vi "QueueRepo.vi"(7 "Action":T1, 8 "error in (no error)":errorcluster, 9 "Event?":bool, 11 "Name":string) -> (0 "error out":errorcluster, 1 "Event?":bool, 2 "queue out":refnum<queue>, 3 "Names":string[](array[string]))   [LabVIEW 2017, in "Communication.lvlib"]
uses:
  Communication.lvlib
  SubVIs/QueueRepo.Action.ctl
  SubVIs/MsgData.ctl
  SubVIs/MsgAck.ctl
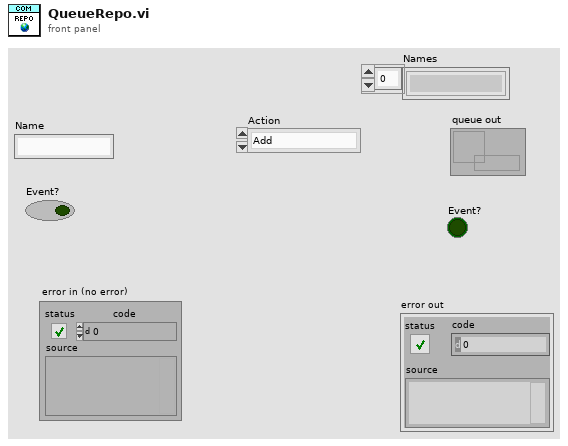
[diagram p1: front panel]
types:
  T1 = typedef "Communication.lvlib/QueueRepo.Action.ctl" = enum16{"Add", "Get", "Destroy", "Get All", "Clear"}
  T2 = typedef "Communication.lvlib/MsgData.ctl" = cluster{"Msg":string, "Data":variant, "Ack":refnum<notifier>}
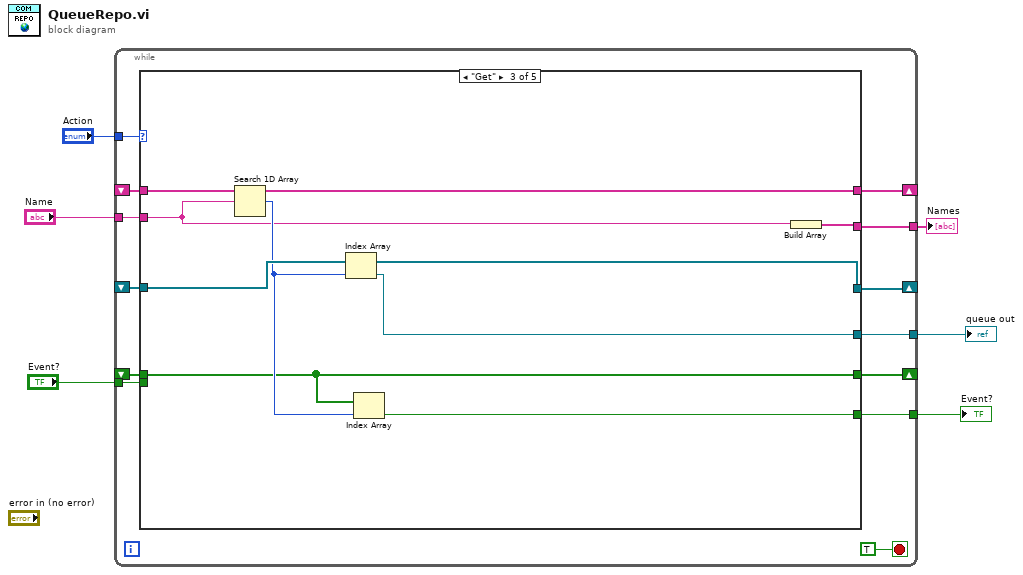
[diagram p0: block diagram]
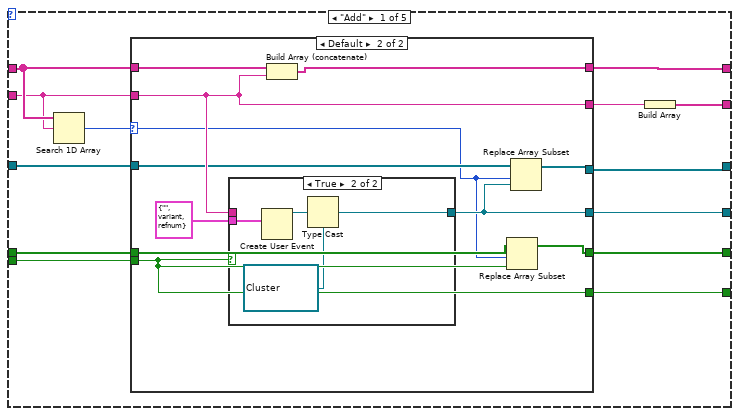
[diagram p2: hidden frame]
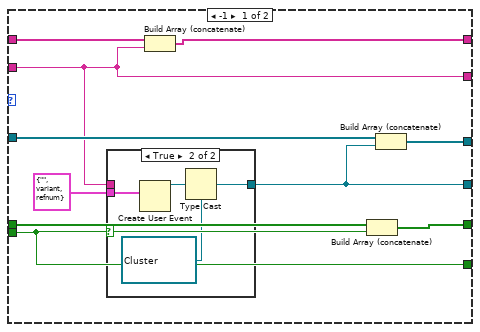
[diagram p3: hidden frame]
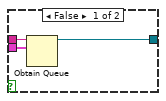
[diagram p4: hidden frame]
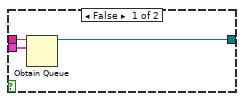
[diagram p5: hidden frame]
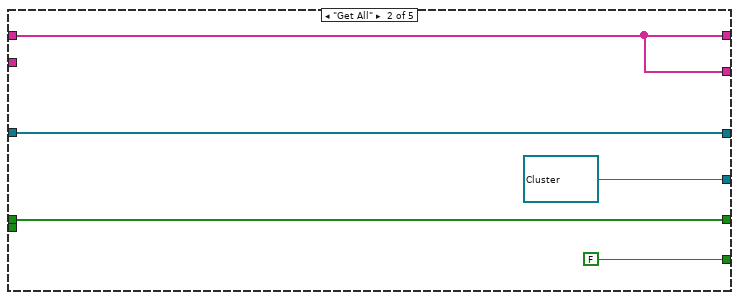
[diagram p6: hidden frame]
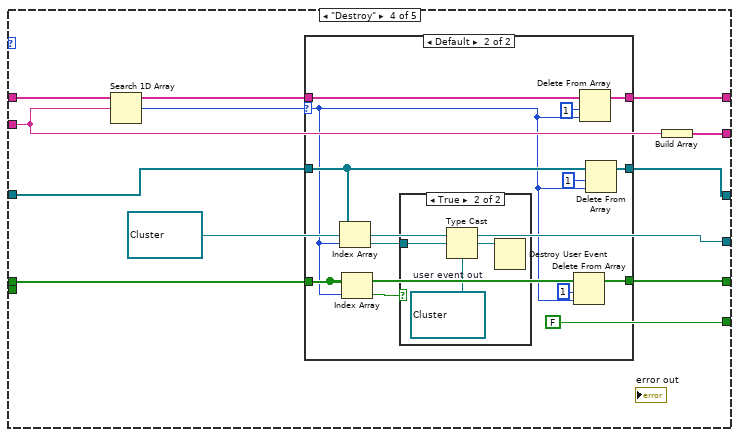
[diagram p7: hidden frame]
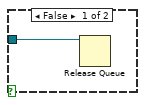
[diagram p9: hidden frame]
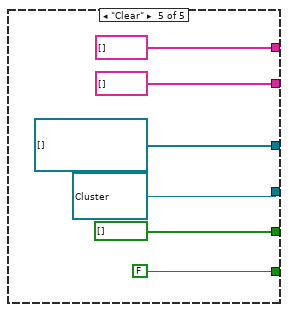
[diagram p10: hidden frame]
diagram:
  n1 = while {
    tunnel: "Action" -> [w19]
    tunnel: "Name" -> [w18]
    shift-right: [w16] -> _
    shift-left: _ -> [w15]
    shift-right: [w14] -> _
    shift-left: _ -> [w13]
    tunnel: [w12] -> w4
    tunnel: "Event?" -> [w11]
    shift-right: [w10] -> _
    shift-left: _ -> [w9]
    tunnel: [w8] -> w2
    tunnel: [w7] -> w1
    stop <- TRUE stop-if-true
    n2 = case shown="\"Get\"" w19 {
      tunnel: w18 -> [w30 _ w73 w84 _]
      tunnel: [w32 w71 w78 w81 string[] []] -> w16
      tunnel: w15 -> [w31 w71 w78 w82 _]
      tunnel: [w29 w72 w79 w90 refnum<queue>[] []] -> w14
      tunnel: w13 -> [w28 w72 w79 w91 _]
      tunnel: [w27 refnum<queue> refnum ("queue out") w80 refnum<queue> refnum ("queue out") refnum<queue> refnum ("queue out")] -> w12
      tunnel: w11 -> [w26 _ _ _ _]
      tunnel: [w25 w69 w76 w86 bool[] []] -> w10
      tunnel: w9 -> [w24 w69 w76 w87 _]
      tunnel: [w23 FALSE ("Event?") w75 FALSE FALSE ("Event?")] -> w8
      tunnel: [w21 w71 w74 w83 string[] []] -> w7
      frame "Add" {
        n3 = Search 1D Array(1D array=w31, element=w30) -> (index of element=w20:i32)  [unwired: 1 in]
        n4 = case shown="Default" w20 {
          selector: w20 -> [_ w51]
          tunnel: [w33 w57] -> w32
          tunnel: w31 -> [w42 w60]
          tunnel: w30 -> [w34 w58]
          tunnel: [w40 w54] -> w29
          tunnel: w28 -> [w39 w56]
          tunnel: [w38 w55] -> w27
          tunnel: w26 -> [w35 w52]
          tunnel: [w37 w50] -> w25
          tunnel: w24 -> [w36 w53]
          tunnel: [w35 w52] -> w23
          tunnel: [w34 w58] -> w22
          frame -1 {
            n5 = case shown="True" w35 {
              tunnel: w34 -> [w45 _]
              tunnel: T2 {"Msg"="", "Data"=variant, "Ack"=refnum} ("Cluster") -> [w44 w49]
              tunnel: [w43 w46] -> w38
              frame False {
                n6 = Obtain Queue(name (unnamed)=w45, element data type=w44) -> (queue out=w43:refnum<queue>)  [unwired: 3 in, 2 out]
              }
              frame True {
                n7 = Create User Event(user event datatype=w49) -> (user event=w48:refnum<user-event>)  [unwired: 1 in, 1 out]
                n8 = Type Cast(type=refnum<queue> refnum ("queue out"), x=w48) -> (*(type *) &x=w46:refnum<queue>)
              }
            }
            n9 = Build Array (concatenate)(w42, w34) -> (w33:string[])
            n10 = Build Array (concatenate)(w36, w35) -> (w37:bool[])
            n11 = Build Array (concatenate)(w39, w38) -> (w40:refnum<queue>[])
          }
          frame Default {
            n12 = case shown="True" w52 {
              tunnel: w58 -> [w63 _]
              tunnel: T2 {"Msg"="", "Data"=variant, "Ack"=refnum} ("Cluster") -> [w62 w67]
              tunnel: [w61 w64] -> w55
              frame False {
                n13 = Obtain Queue(name (unnamed)=w63, element data type=w62) -> (queue out=w61:refnum<queue>)  [unwired: 3 in, 2 out]
              }
              frame True {
                n14 = Create User Event(user event datatype=w67) -> (user event=w66:refnum<user-event>)  [unwired: 1 in, 1 out]
                n15 = Type Cast(type=refnum<queue> refnum ("queue out"), x=w66) -> (*(type *) &x=w64:refnum<queue>)
              }
            }
            n16 = Build Array (concatenate)(w60, w58) -> (w57:string[])
            n17 = Replace Array Subset(array=w53, new element=w52, index=w51) -> (w50:bool[])
            n18 = Replace Array Subset(array=w56, new element=w55, index=w51) -> (w54:refnum<queue>[])
          }
        }
        n19 = Build Array(w22) -> (w21:string[])
      }
      frame "Get All" {
      }
      frame "Get" {
        n20 = Search 1D Array(1D array=w78, element=w73) -> (index of element=w77:i32)  [unwired: 1 in]
        n21 = Index Array(array=w79, index=w77) -> (element=w80:refnum<queue>)
        n22 = Index Array(array=w76, index=w77) -> (element=w75:bool)
        n23 = Build Array(w73) -> (w74:string[])
      }
      frame "Destroy" {
        n24 = Search 1D Array(1D array=w82, element=w84) -> (index of element=w88:i32)  [unwired: 1 in]
        n25 = case shown="Default" w88 {
          selector: w88 -> [_ w95]
          tunnel: w91 -> [w94 w105]
          tunnel: [w94 w104] -> w90
          tunnel: w87 -> [w93 w101]
          tunnel: [w93 w100] -> w86
          tunnel: w82 -> [w92 w98]
          tunnel: [w92 w97] -> w81
          frame -1 {
          }
          frame Default {
            n26 = Index Array(array=w105, index=w95) -> (element=w106:refnum<queue>)
            n27 = Index Array(array=w101, index=w95) -> (element=w102:bool)
            n28 = case shown="True" w102 {
              tunnel: w106 -> [w107 w110]
              frame False {
                n29 = Release Queue(queue=w107) -> ()  [unwired: 2 in, 3 out]
              }
              frame True {
                w109 = refnum<user-event> refnum  # user event out
                n30 = Type Cast(type=w109, x=w110) -> (*(type *) &x=w108:refnum<user-event>)
                n31 = Destroy User Event(user event=w108) -> ()  [unwired: 1 in, 1 out]
              }
            }
            n32 = Delete From Array(array=w101, length=1, index=w95) -> (array with subset deleted=w100:bool[])  [unwired: 1 out]
            n33 = Delete From Array(array=w98, length=1, index=w95) -> (array with subset deleted=w97:string[])  [unwired: 1 out]
            n34 = Delete From Array(array=w105, length=1, index=w95) -> (array with subset deleted=w104:refnum<queue>[])  [unwired: 1 out]
          }
        }
        n35 = Build Array(w84) -> (w83:string[])
      }
      frame "Clear" {
      }
    }
  }
  "queue out" <- w4
  "Event?" <- w2
  "Names" <- w1
